vi "util_array_to_string.vi"(0 "Header":string, 1 "Format":string, 2 "Input 1D array":dbl[](array[numeric]), 3 "Unit":string) -> (7 "Output 1D array":string[](array[string]))   [LabVIEW 2016]
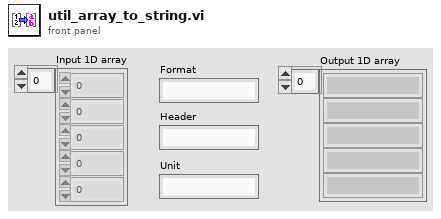
[diagram p1: front panel]
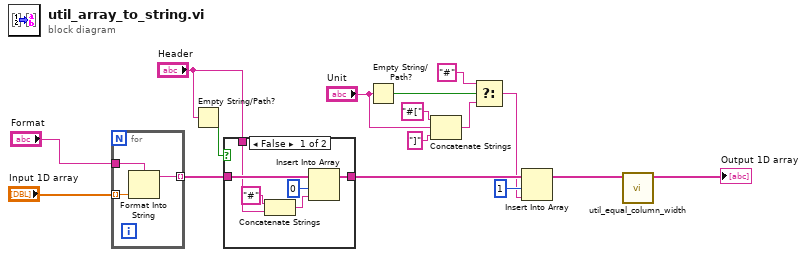
[diagram p0: block diagram]
diagram:
  n1 = for {
    tunnel: "Input 1D array" -> [w19] mode=indexing
    tunnel: "Format" -> [w18]
    tunnel: [w17] -> w14 mode=indexing
    n2 = Format Into String(format string=w18, w19) -> (resulting string=w17:string)  [unwired: 2 in, 1 out]
  }
  n3 = Empty String/Path?(string/path="Header") -> (empty?=w13:bool)
  n4 = case shown="False" w13 {
    tunnel: w14 -> [w25 w26]
    tunnel: "Header" -> [w21 _]
    tunnel: [w23 w26] -> w12
    frame False {
      n5 = Concatenate Strings("#" ("string"), w21) -> (w20:string)
      n6 = Insert Into Array(array=w25, index=0, new element=w20) -> (w23:string[])
    }
    frame True {
    }
  }
  n7 = Empty String/Path?(string/path="Unit") -> (empty?=w8:bool)
  n8 = Concatenate Strings("#[" ("string"), "Unit", "]" ("string")) -> (w6:string)
  n9 = Select(t="#" ("string"), s=w8, f=w6) -> (s? t:f=w4:string)
  n10 = Insert Into Array(array=w12, index=1, new element=w4) -> (w2:string[])
  n11 = call "util_equal_column_width.vi"("Input 1D array"=w2) -> ("Output 1D array"=→"Output 1D array":string[])  [unwired: 10 in]
